vi "MM6Archiver.open file.vi"(0 "i ref in":refnum<vi>, 3 "ms timeout (10000)":i32=10000, 5 "error in (no error)":errorcluster) -> (14 "i ref out":refnum<vi>, 17 "timed out":bool, 19 "error out":errorcluster)   [LabVIEW 2014, in "MM6Archiver.lvlib"]
doc: "Opens a new file. The file name is composed by the file prefix only. If the file already exists, it will NOT be replaced."
uses:
  MM6Archiver.lvlib
  CSData/DiscArchiver/DiscArchiver.lvlib
  CSlibraries-extern/DimLVEvent/LVDimInterface/LVDimInterface.lvlib
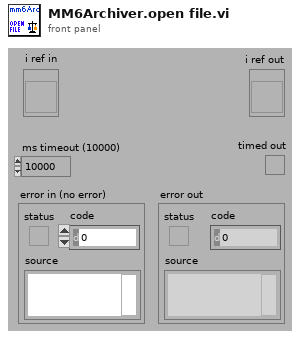
[diagram p1: front panel]
types:
  T1 = enum16{"open", "replace", "create", "open or create", "replace or create", "replace or create with confirmation"}
  T2 = typedef "DiscArchiver.lvlib/DiscArchiver.i attribute.ctl" = cluster{"file prefix":string, "actual file":string, "nOfEvents":i32, "file":refnum<file>, "eventBuilder":string, "disc size alarm":bool, "dataDescription":string, "dataDescriptionURL":string, "eventDataURL":string, "headerID":dbl, "completeData":bool, "nOfEventsID":i32, "dataFileID":i32}
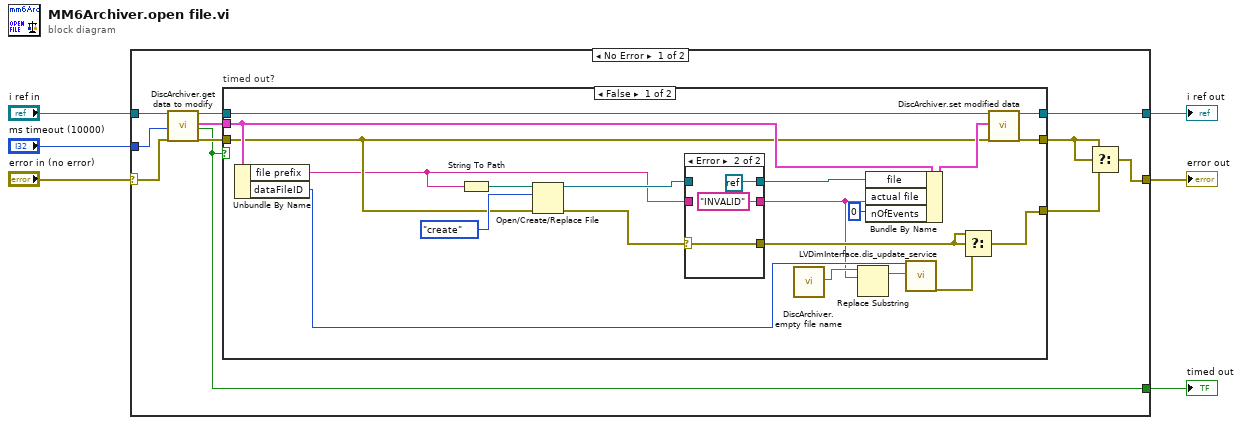
[diagram p0: block diagram]
diagram:
  n1 = case shown="No Error" "error in (no error)" {
    selector: "error in (no error)" -> [w7 w46]
    tunnel: "i ref in" -> [w17 w47]
    tunnel: [w16 w47] -> w5
    tunnel: "ms timeout (10000)" -> [w12 _]
    tunnel: [w11 _] -> w3
    tunnel: [w8 w46] -> w2
    frame No Error {
      n2 = call "DiscArchiver.get data to modify.vi"("i ref in"=w17, "ms timeout (10000)"=w12, "error in (no error)"=w7) -> ("i ref out"=w15:refnum<vi>, "i attribute"=w13:T2, "timed out"=w11:bool, "error out"=w14:errorcluster)  [unwired: 13 in]
      n3 = case "timed out?" shown="False" w11 {
        tunnel: [w37 w44] -> w10
        tunnel: [w36 w45] -> w16
        tunnel: w15 -> [w35 w45]
        tunnel: w14 -> [w29 w44]
        tunnel: w13 -> [w34 _]
        tunnel: [w24 w44] -> w9
        frame False {
          n4 = Unbundle By Name(w34) -> ("file prefix"=w18:string, "dataFileID"=w32:i32)
          n5 = String To Path(string=w18) -> (path=w31:path)
          n6 = Open/Create/Replace File(file path (use dialog)=w31, error in=w29, operation (0:open)=T1."create") -> (refnum out=w20:refnum<file>, error out=w23:errorcluster)  [unwired: 3 in, 1 out]
          n7 = case shown="Error" w23 {
            selector: w23 -> [w40 w41]
            tunnel: [w40 w41] -> w22
            tunnel: [w39 refnum<k0> refnum] -> w21
            tunnel: w20 -> [w39 _]
            tunnel: [w38 "INVALID" ("file prefix")] -> w19
            tunnel: w18 -> [w38 _]
            frame No Error {
            }
            frame Error {
            }
          }
          n8 = call "DiscArchiver.empty file name.vi"() -> ("emptyString"=w26:string)  [unwired: 19 in]
          n9 = Replace Substring(4:w19, 5:w26) -> (1:w27:string)  [unwired: 2 in, 1 out]
          n10 = Bundle By Name(cluster=w34, "file"=w21, "actual file"=w19, "nOfEvents"=0 ("# of items")) -> (w33:T2)
          n11 = call "LVDimInterface.dis_update_service.vi"("my_serviceID"=w32, "data"=w27) -> ("error out"=w25:errorcluster)  [unwired: 15 in, 2 out]
          n12 = Select(t=w22, s=w22, f=w25) -> (s? t:f=w24:errorcluster)
          n13 = call "DiscArchiver.set modified data.vi"("i ref in"=w35, "i attribute"=w33, "error in (no error)"=w29) -> ("i ref out"=w36:refnum<vi>, "error out"=w37:errorcluster)  [unwired: 15 in]
        }
        frame True {
        }
      }
      n14 = Select(t=w10, s=w10, f=w9) -> (s? t:f=w8:errorcluster)
    }
    frame Error {
    }
  }
  "error out" <- w2
  "i ref out" <- w5
  "timed out" <- w3
